vi "Create Preview Tree.vi"(8 "error in (no error)":errorcluster, 11 "Summary":refnum<vi>) -> (0 "error out":errorcluster)   [LabVIEW 2017, in "WebServiceImporter.lvlib" / "Main Panel.lvlib" / "Preview.lvlib"]
uses:
  <vilib>/Platform/WebService/Main Panel/Pages/Preview/Preview.lvlib
  <vilib>/Platform/WebService/Global/Const Strings.vi
  <vilib>/Platform/WebService/ProxyDll Generator/ProxyDll Generator.lvlib
  <vilib>/Platform/WebService/VI Generator/VI Generator.lvlib
  <vilib>/Platform/WebService/WebServiceImporter.lvlib
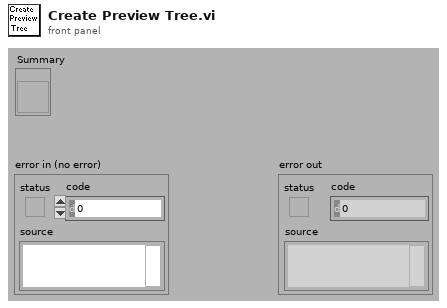
[diagram p1: front panel]
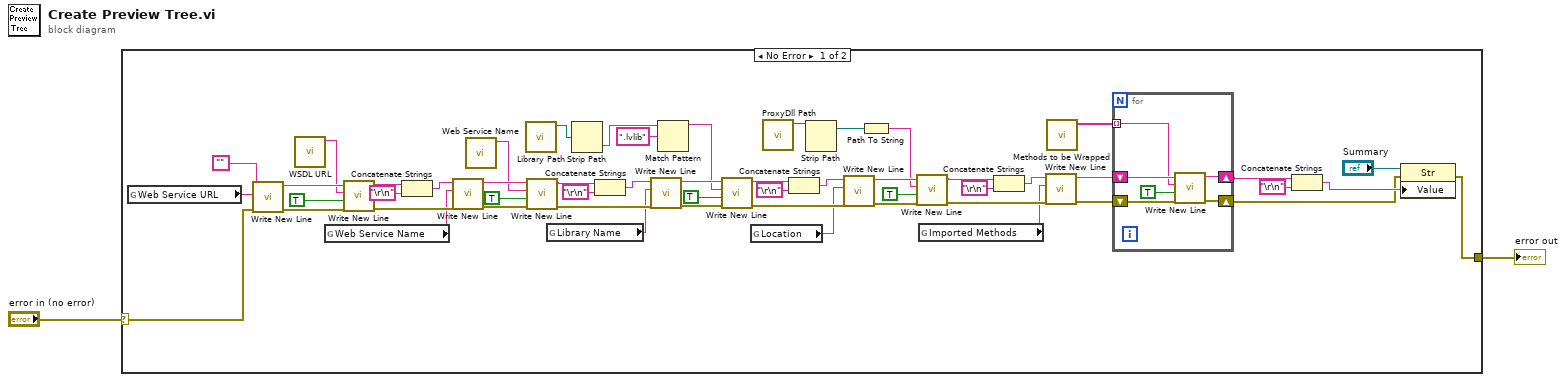
[diagram p0: block diagram]
diagram:
  n1 = case shown="No Error" "error in (no error)" {
    selector: "error in (no error)" -> [w47 w62]
    tunnel: [w48 w62] -> w1
    frame No Error {
      n2 = global read "Const Strings.vi" "Web Service URL"() -> (w44:string)
      n3 = call <vilib>:"Write New Line.vi"("error in (no error)"=w47, "New Line"=w44, "Text"="") -> ("error out"=w46:errorcluster, "Text (out)"=w45:string)  [unwired: 7 in]
      n4 = call <vilib>:"WSDL URL.vi"() -> ("WSDL URL (out)"=w41:string)  [unwired: 10 in, 1 out]
      n5 = global read "Const Strings.vi" "Web Service Name"() -> (w36:string)
      n6 = call <vilib>:"Write New Line.vi"("error in (no error)"=w46, "Indent ? ( F)"=TRUE, "New Line"=w41, "Text"=w45) -> ("error out"=w38:errorcluster, "Text (out)"=w40:string)  [unwired: 6 in]
      n7 = Concatenate Strings(w40, "\r\n") -> (w37:string)
      n8 = call <vilib>:"Write New Line.vi"("error in (no error)"=w38, "New Line"=w36, "Text"=w37) -> ("error out"=w35:errorcluster, "Text (out)"=w34:string)  [unwired: 7 in]
      n9 = call <vilib>:"Web Service Name.vi"() -> ("Web Service Name (out)"=w32:string)  [unwired: 10 in, 1 out]
      n10 = call <vilib>:"Library Path.vi"() -> ("Path (out)"=w52:path)  [unwired: 10 in, 1 out]
      n11 = call <vilib>:"Write New Line.vi"("error in (no error)"=w35, "Indent ? ( F)"=TRUE, "New Line"=w32, "Text"=w34) -> ("error out"=w28:errorcluster, "Text (out)"=w30:string)  [unwired: 6 in]
      n12 = global read "Const Strings.vi" "Library Name"() -> (w27:string)
      n13 = Strip Path(path=w52) -> (name=w51:string)  [unwired: 1 out]
      n14 = Concatenate Strings(w30, "\r\n") -> (w29:string)
      n15 = call <vilib>:"Write New Line.vi"("error in (no error)"=w28, "New Line"=w27, "Text"=w29) -> ("error out"=w26:errorcluster, "Text (out)"=w25:string)  [unwired: 7 in]
      n16 = Match Pattern(string=w51, regular expression=".lvlib") -> (before substring=w23:string)  [unwired: 1 in, 3 out]
      n17 = call <vilib>:"Write New Line.vi"("error in (no error)"=w26, "Indent ? ( F)"=TRUE, "New Line"=w23, "Text"=w25) -> ("error out"=w19:errorcluster, "Text (out)"=w21:string)  [unwired: 6 in]
      n18 = global read "Const Strings.vi" "Location"() -> (w18:string)
      n19 = call <vilib>:"ProxyDll Path.vi"() -> ("ProxyDll Path (out)"=w54:path)  [unwired: 10 in, 1 out]
      n20 = Concatenate Strings(w21, "\r\n") -> (w20:string)
      n21 = Strip Path(path=w54) -> (stripped path=w53:path)  [unwired: 1 out]
      n22 = call <vilib>:"Write New Line.vi"("error in (no error)"=w19, "New Line"=w18, "Text"=w20) -> ("error out"=w17:errorcluster, "Text (out)"=w15:string)  [unwired: 7 in]
      n23 = Path To String(path=w53) -> (string=w14:string)
      n24 = call <vilib>:"Write New Line.vi"("error in (no error)"=w17, "Indent ? ( F)"=TRUE, "New Line"=w14, "Text"=w15) -> ("error out"=w10:errorcluster, "Text (out)"=w12:string)  [unwired: 6 in]
      n25 = global read "Const Strings.vi" "Imported Methods"() -> (w9:string)
      n26 = Concatenate Strings(w12, "\r\n") -> (w11:string)
      n27 = call <vilib>:"Write New Line.vi"("error in (no error)"=w10, "New Line"=w9, "Text"=w11) -> ("error out"=w8:errorcluster, "Text (out)"=w7:string)  [unwired: 7 in]
      n28 = call <vilib>:"Methods to be Wrapped.vi"() -> ("Methods to be Wrapped (out)"=w55:string[])  [unwired: 10 in, 1 out]
      n29 = for {
        tunnel: w55 -> [w58] mode=indexing
        shift-right: [w56] -> w5
        shift-left: w7 -> [w61]
        shift-right: [w57] -> w3
        shift-left: w8 -> [w60]
        n30 = call <vilib>:"Write New Line.vi"("error in (no error)"=w60, "Indent ? ( F)"=TRUE, "New Line"=w58, "Text"=w61) -> ("error out"=w57:errorcluster, "Text (out)"=w56:string)  [unwired: 6 in]
      }
      n31 = Concatenate Strings(w5, "\r\n") -> (w4:string)
      n32 = property class="Str"(reference="Summary", error in=w3, "Value"=w4) -> (error out=w48:errorcluster)  [unwired: 1 out]
    }
    frame Error {
    }
  }
  "error out" <- w1
